vi "BRig_Host__Loop_Consumer_RunState__loadData.vi"(10 "input_dataLC":u16[](array[numeric]), 11 "input_dataExp":u16[](array[numeric])) -> (2 "output_dataLC":u16[](array[numeric]), 3 "output_dataExp":u16[](array[numeric]))   [LabVIEW 2014]
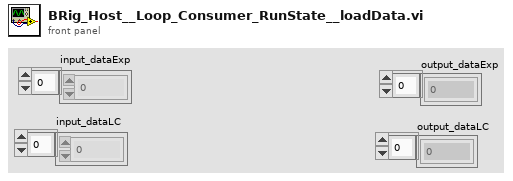
[diagram p1: front panel]
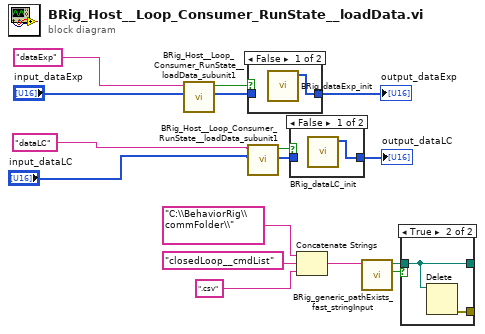
[diagram p0: block diagram]
diagram:
  n1 = call "BRig_Host__Loop_Consumer_RunState__loadData_subunit1.vi"("input_data"="input_dataExp", "input_name"="dataExp" ("string")) -> (2:"output_data"=w12:u16[], 3:"output_data"=w11:bool)  [unwired: 8 in]
  n2 = case shown="False" w11 {
    tunnel: w12 -> [_ w18]
    tunnel: [w17 w18] -> w10
    frame False {
      n3 = call "BRig_dataExp_init.vi"() -> ("output_dataExp"=w17:u16[])  [unwired: 11 in]
    }
    frame True {
    }
  }
  "output_dataExp" <- w10
  n4 = call "BRig_Host__Loop_Consumer_RunState__loadData_subunit1.vi"("input_data"="input_dataLC", "input_name"="dataLC" ("string")) -> (2:"output_data"=w9:u16[], 3:"output_data"=w8:bool)  [unwired: 8 in]
  n5 = case shown="False" w8 {
    tunnel: w9 -> [_ w20]
    tunnel: [w19 w20] -> w7
    frame False {
      n6 = call "BRig_dataLC_init.vi"() -> ("output_dataLC"=w19:u16[])  [unwired: 11 in]
    }
    frame True {
    }
  }
  "output_dataLC" <- w7
  n7 = Concatenate Strings("C:\\BehaviorRig\\commFolder\\", "closedLoop__cmdList" ("string"), ".csv" ("string")) -> (w1:string)
  n8 = call "BRig_generic_pathExists_fast_stringInput.vi"("input_filePath"=w1) -> ("output_Iexist"=w3:bool, "output_filePath"=w2:path)  [unwired: 8 in, 1 out]
  n9 = case shown="True" w3 {
    tunnel: w2 -> [w21 w22]
    tunnel: [_ w23] -> _
    tunnel: [w21 w22] -> _
    frame False {
    }
    frame True {
      n10 = Delete(path (use dialog)=w22) -> (error out=w23:errorcluster)  [unwired: 4 in, 2 out]
    }
  }
